vi "lorem_ipsum.vi"(7 "start with 'lorem ipsum...' (T)":bool=TRUE, 8 "paragraph delimiter (2x CR)":string="\n\n", 9 "mode (paragraphs)":enum16{"paragraphs", "words", "characters"}(ring), 10 "N (5)":i32=5) -> (2 "lorem ipsum":string)   [LabVIEW 2015]
uses:
  <vilib>/Analysis/1siggen.llb/Riffle Array (I32).vi
  <userlib>/_OpenG.lib/array/array.llb/Index 1D Array Elements (String)__ogtk.vi
  <vilib>/Analysis/NI_AALBase.lvlib
panel:
  # "Based on https://www.lipsum.com"
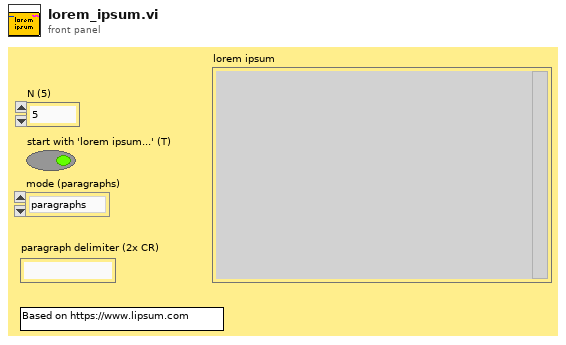
[diagram p1: front panel]
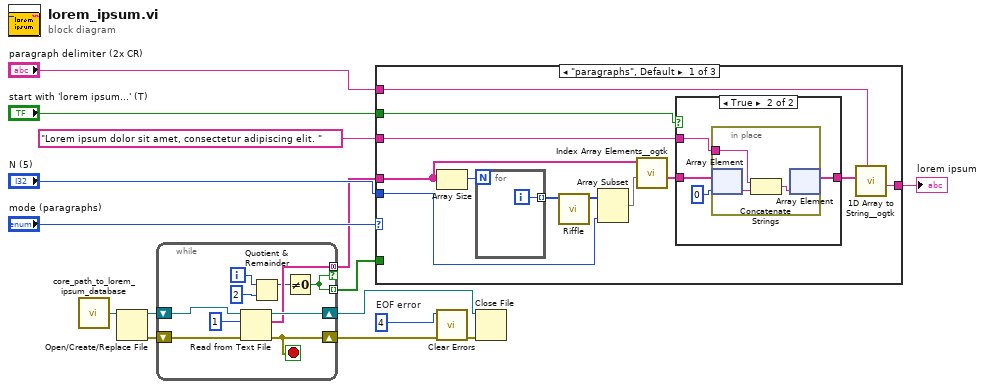
[diagram p0: block diagram]
diagram:
  w2 = 4  # EOF error
  n1 = call "core_path_to_lorem_ipsum_database.vi"() -> ("path to database"=w15:path)
  n2 = Open/Create/Replace File(file path (use dialog)=w15) -> (refnum out=w12:refnum<file>, error out=w13:errorcluster)  [unwired: 5 in, 1 out]
  n3 = while {
    tunnel: [w21] -> w5 mode=concatenating if=w17
    shift-right: [w18] -> w4
    shift-left: w13 -> [w24]
    shift-right: [w25] -> w14
    shift-left: w12 -> [w23]
    tunnel: [w17] -> w1 mode=indexing
    i -> [w20]
    stop <- w18 stop-if-true
    n4 = Read from Text File(file (use dialog)=w23, count=1, error in=w24) -> (refnum out=w25:refnum<file>, text=w21:string[], error out=w18:errorcluster)  [unwired: 1 in, 1 out]
    n5 = Quotient & Remainder(x=w20, y=2) -> (x-y*floor(x/y)=w16:i32)  [unwired: 1 out]
    n6 = Not Equal To 0?(x=w16) -> (x != 0?=w17:bool)
  }
  n7 = case shown="\"paragraphs\", Default" "mode (paragraphs)" {
    tunnel: w5 -> [w33 _ _]
    tunnel: "N (5)" -> [w34 _ _]
    tunnel: "start with 'lorem ipsum...' (T)" -> [w31 _ _]
    tunnel: "Lorem ipsum dolor sit amet, consectetur adipiscing elit. " -> [w30 _ _]
    tunnel: [w27 _ _] -> w7
    tunnel: "paragraph delimiter (2x CR)" -> [w26 _ _]
    tunnel: w1 -> [_ _ _]
    frame "paragraphs", Default {
      n8 = Array Size(array=w33) -> (size(s)=w37:i32)
      n9 = for {
        N: w37 -> [_]
        tunnel: [w46] -> w36 mode=indexing
        i -> [w46]
      }
      n10 = call-poly <vilib>:"Riffle.vi"("X"=w36) -> ("Riffled {X}"=w35:i32[])  [unwired: 8 in, 2 out]
      n11 = Array Subset(array=w35, length=w34) -> (w32:i32[])  [unwired: 1 in]
      n12 = call-poly <userlib>:"Index Array Elements__ogtk.vi"("indices"=w32, "array"=w33) -> ("elements"=w29:string[])  [unwired: 9 in]
      n13 = case shown="True" w31 {
        tunnel: w30 -> [_ w42]
        tunnel: w29 -> [w38 w41]
        tunnel: [w38 w40] -> w28
        frame False {
        }
        frame True {
          n14 = in-place {
            in-place-border: w42 -> [w43]
            n15 = in-place-array #1(w41, 0) -> (w45:string)
            n16 = Concatenate Strings(w43, w45) -> (w44:string)
            n17 = in-place-array #1(w44) -> (w40:string[])  [unwired: 1 out]
          }
        }
      }
      n18 = call <userlib>:"1D Array to String__ogtk.vi"("delimiter (Tab)"=w26, "Array of Strings"=w28) -> ("delimited string"=w27:string)  [unwired: 9 in]
    }
    frame "words" {
      # "WIP"
    }
    frame "characters" {
      # "WIP"
    }
  }
  "lorem ipsum" <- w7
  n19 = call <vilib>:"Clear Errors.vi"("error in (no error)"=w4, "specific error code to clear (0: all)"=w2) -> ("error out"=w3:errorcluster)  [unwired: 4 in, 1 out]
  n20 = Close File(refnum=w14, error in=w3) -> ()  [unwired: 2 out]
